vi "Read KeyProperties.vi"(8 "error in (no error)":errorcluster, 11 "TypeMap in":refnum<class "TypeMap.lvclass">) -> (0 "error out":errorcluster, 2 "KeyProperties":string[](array[string])=["Id"], 3 "TypeMap out":refnum<class "TypeMap.lvclass">)   [LabVIEW 2020, in "ORM.lvlib" / "TypeMap.lvclass"]
uses:
  TypeMap.lvclass
  TypeMap.lvclass/TypeMap.ctl
  Read Autokey.vi
  Read ExcludeIDFromKeyProp.vi
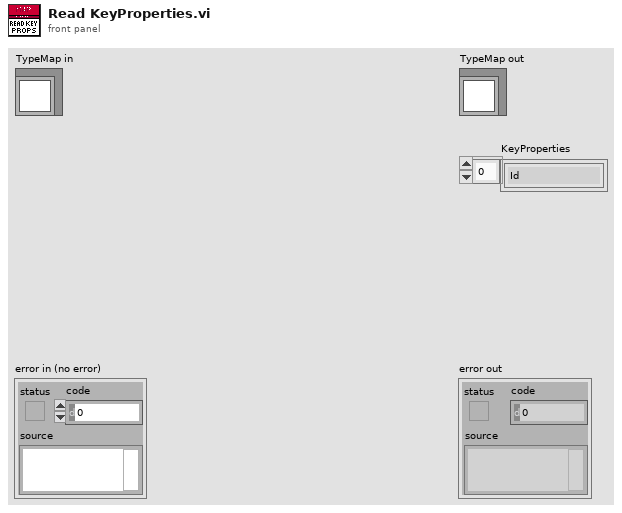
[diagram p1: front panel]
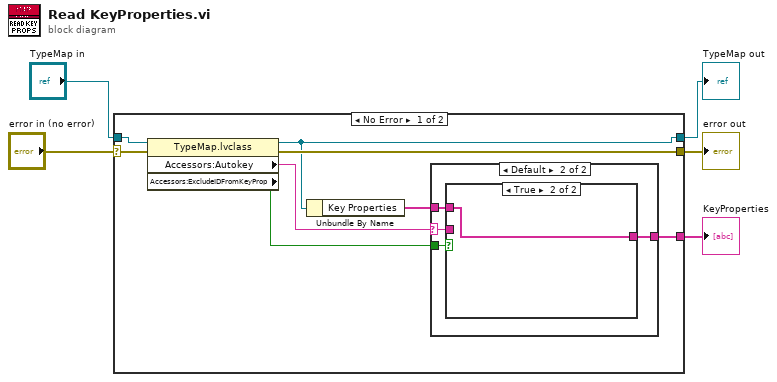
[diagram p0: block diagram]
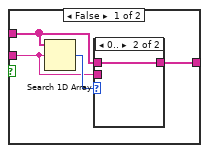
[diagram p3: hidden frame]
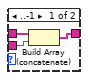
[diagram p4: hidden frame]
diagram:
  n1 = case shown="No Error" "error in (no error)" {
    selector: "error in (no error)" -> [w9 w28]
    tunnel: [w8 w28] -> w4
    tunnel: [w7 w29] -> w2
    tunnel: "TypeMap in" -> [w11 w29]
    tunnel: [w12 _] -> w1
    frame No Error {
      n2 = property class="TypeMap.lvclass"(reference=w11, error in=w9) -> (reference out=w7:refnum<class "TypeMap.lvclass">, error out=w8:errorcluster, "Accessors:Autokey"=w10:string, "Accessors:ExcludeIDFromKeyProp"=w6:bool)
      n3 = Unbundle By Name(w7) -> ("Key Properties"=w13:string[])
      n4 = case shown="Default" w10 {
        selector: w10 -> [_ w16]
        tunnel: w13 -> [w14 w18]
        tunnel: [w14 w17] -> w12
        tunnel: w6 -> [_ w15]
        frame "" {
        }
        frame Default {
          n5 = case shown="True" w15 {
            tunnel: w18 -> [w22 w27]
            tunnel: [w21 w27] -> w17
            tunnel: w16 -> [w19 _]
            frame False {
              n6 = Search 1D Array(1D array=w22, element=w19) -> (index of element=w20:i32)  [unwired: 1 in]
              n7 = case shown="0.." w20 {
                tunnel: w22 -> [w24 w26]
                tunnel: [w23 w26] -> w21
                tunnel: w19 -> [w25 _]
                frame ..-1 {
                  n8 = Build Array (concatenate)(w24, w25) -> (w23:string[])
                }
                frame 0.. {
                }
              }
            }
            frame True {
            }
          }
        }
      }
    }
    frame Error {
    }
  }
  "error out" <- w4
  "TypeMap out" <- w2
  "KeyProperties" <- w1
